vi "20T_CS_schleife_init.vi"   [LabVIEW 2016]
uses:
  Monitors/Utility/Monitor Communication/Gustav/20T_Control.ctl
  Global/Global Variables/global.vi
  Global/Global Variables/Data_Display_global.vi
  Monitors/Utility/Monitor Communication/sub-vis/20T_Open_Queue.vi
  Monitors/Utility/Monitor Communication/sub-vis/20T_Queue_Commands.vi
  Instrument_Setup.vi
types:
  T1 = typedef "20T_Control.ctl" = cluster{"Clamp":bool, "Switch Heater":bool, "Go to Zero":bool, "Go to Set":bool, "Go to Hold":bool, "Setpoint (T)":dbl, "Rate (T/min)":dbl, "Set Rate":bool}
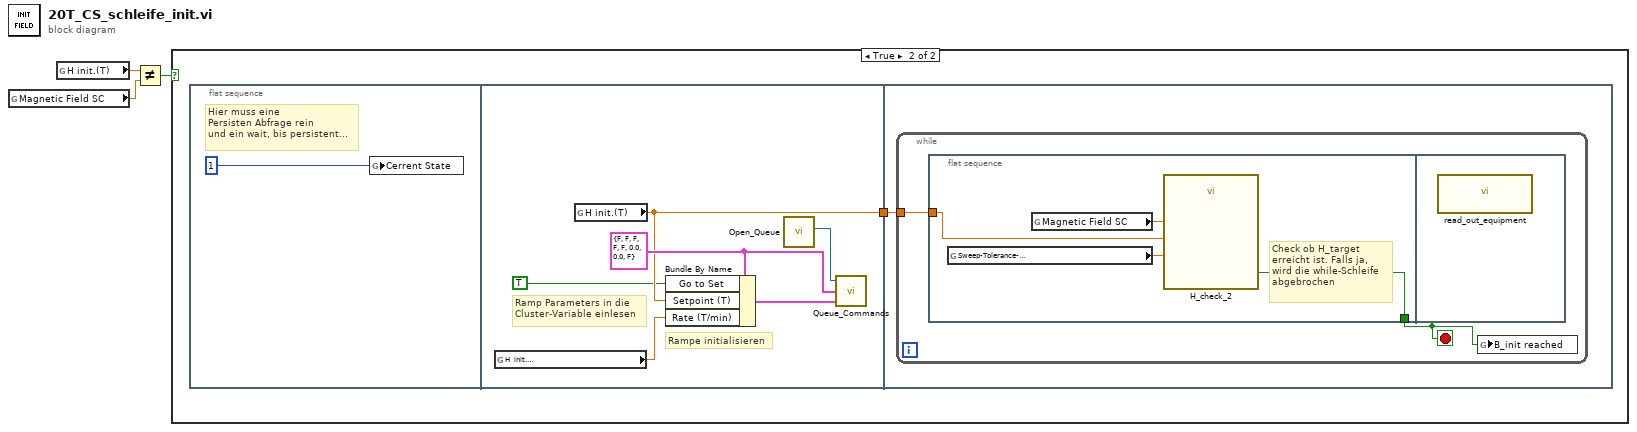
[diagram p0: block diagram]
diagram:
  n1 = global read "Data_Display_global.vi" "Magnetic Field SC"() -> (w2:dbl)
  n2 = global read "global.vi" "H init.(T)"() -> (w3:dbl)
  n3 = Not Equal?(x=w3, y=w2) -> (x != y?=w1:bool)
  n4 = case shown="True" w1 {
    frame False {
    }
    frame True {
      n5 = flat-sequence {
        tunnel: [w9] -> w4
        tunnel: w4 -> [w12]
        frame #0 {
          # "Hier muss eine \nPersisten Abfrage rein\nund ein wait, bis persistent..."
          n6 = global write "global.vi" "Cerrent State"(1) -> ()
        }
        frame #1 {
          w10 = T1 {"Clamp"=FALSE, "Switch Heater"=FALSE, "Go to Zero"=FALSE, "Go to Set"=FALSE, "Go to Hold"=FALSE, "Setpoint (T)"=0.0, "Rate (T/min)"=0.0, "Set Rate"=FALSE} ("Last Status")
          # "Rampe initialisieren"
          # "Ramp Parameters in die \nCluster-Variable einlesen"
          n7 = global read "global.vi" "H  init. \nGeschw.(T/min)"() -> (w8:dbl)
          n8 = global read "global.vi" "H init.(T)"() -> (w9:dbl)
          n9 = Bundle By Name(cluster=w10, "Go to Set"=TRUE, "Setpoint (T)"=w9, "Rate (T/min)"=w8) -> (w7:T1)
          n10 = call-poly "Open_Queue.vi"() -> ("queue out"=w11:refnum<queue>)  [unwired: 10 in, 1 out]
          n11 = call-poly "Queue_Commands.vi"("20 T Control"=w7, "Last Status"=w10, "20T Queue"=w11) -> ()  [unwired: 1 out]
        }
        frame #2 {
          n12 = while {
            tunnel: w12 -> [w13]
            stop <- w14 stop-if-true
            n13 = flat-sequence {
              tunnel: [w18] -> w14
              tunnel: w13 -> [w16]
              frame #0 {
                # "Check ob H_target\nerreicht ist. Falls ja,\nwird die while-Schleife\nabgebrochen"
                n14 = global read "Instrument_Setup.vi" "Sweep-Tolerance-\nMagnetic-Field"() -> (w17:dbl)
                n15 = global read "Data_Display_global.vi" "Magnetic Field SC"() -> (w15:dbl)
                n16 = call "H_check_2.vi"("Sweep\nTolerance %"=w17, "H_in"=w15, "H_target (K)"=w16) -> ("= H target"=w18:bool)  [unwired: 8 in]
              }
              frame #1 {
                n17 = call "read_out_equipment.vi"() -> ()  [unwired: 1 in]
              }
            }
            n18 = global write "Data_Display_global.vi" "B_init reached"(w14) -> ()
          }
        }
      }
    }
  }
